vi "Create Citadel Query Trace Data String.vi"(5 "End Time String":string, 7 "Start Time String":string, 8 "error in":errorcluster, 9 "db Path":string, 10 "Trace Name":string, 11 "Server":string) -> (0 "error out":errorcluster, 3 "GET string":string)   [LabVIEW 2019]
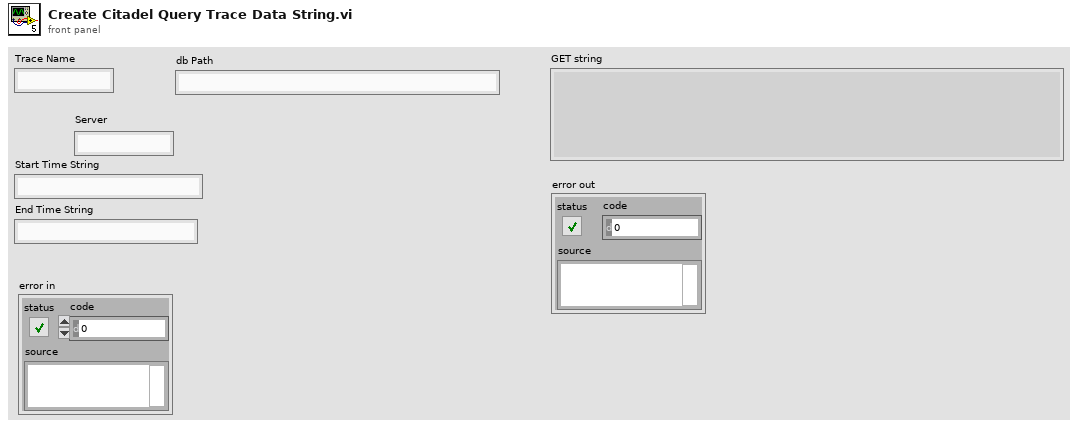
[diagram p1: front panel]
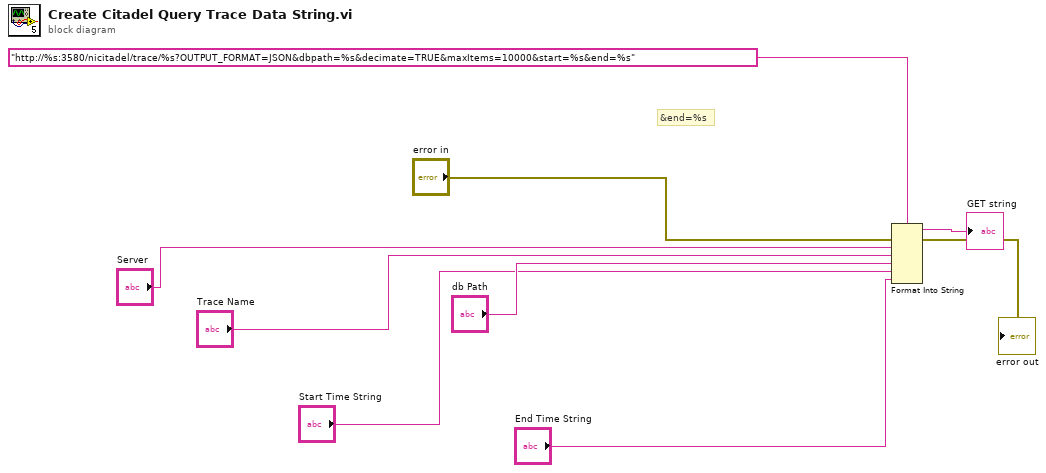
[diagram p0: block diagram]
diagram:
  # "&end=%s"
  n1 = Format Into String(format string="http://%s:3580/nicitadel/trace/%s?OUTPUT_FORMAT=JSON&dbpath=%s&decimate=TRUE&maxItems=10000&start=%s&end=%s", error in="error in", "Server", "Trace Name", "db Path", "Start Time String", "End Time String") -> (resulting string=→"GET string":string, error out=→"error out":errorcluster)  [unwired: 1 in]
